vi "Example - Building a Source Distribution.vi"() -> ()   [LabVIEW 2020]
doc: "Demonstrates the use of the Application Builder API to create and build a Source Distribution build specification."
uses:
  <vilib>/AppBuilder/AB_API/common/AB_API Version Number.ctl
  <vilib>/AppBuilder/AB_API/SDIST/NI_AB_API_SDIST.lvclass
panel:
  out "Generated Files":path[](array[path])
  # "Overview: Demonstrates the use of the Application Builder API to create and build a Source Distribution build specification.\nRequirements: LabVIEW Professional Development System or LabVIEW Application Builder\nInstructions:\n1. Run the VI. A Source Distribution build specification will be created, which will then be built programmatically.\n2. Examine the SDIST build specification in the new project.\n3. Close the temporary project and delete the temporary project files generated by this example when you are done."
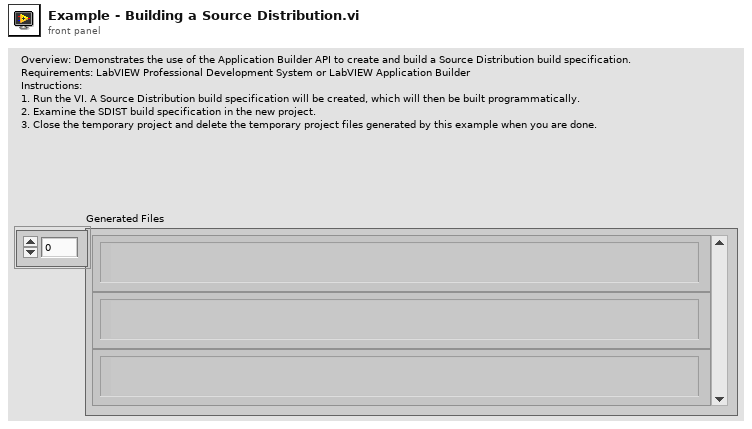
[diagram p1: front panel]
types:
  T1 = typedef "AB_API Version Number.ctl" = cluster{"Major":u16, "Minor":u16, "Fix":u16, "Build":u16}
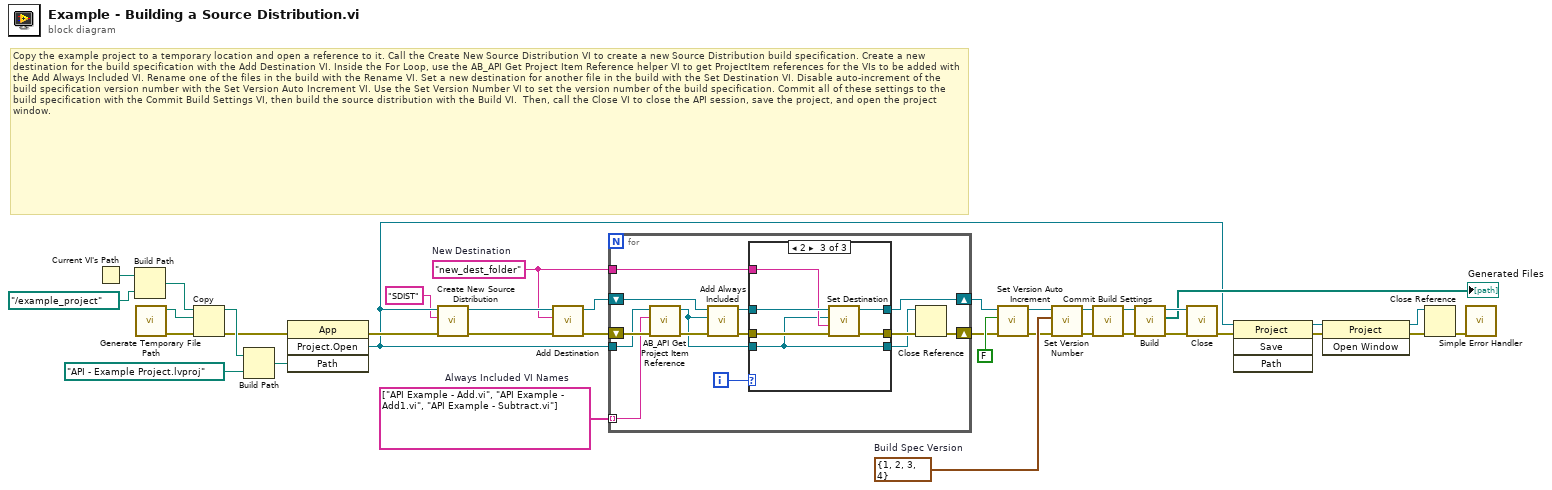
[diagram p0: block diagram]
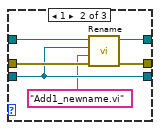
[diagram p3: hidden frame]
diagram:
  w4 = "new_dest_folder"  # New Destination
  w15 = T1 {"Major"=1, "Minor"=2, "Fix"=3, "Build"=4}  # Build Spec Version
  w31 = string[] ["API Example - Add.vi", "API Example - Add1.vi", "API Example - Subtract.vi"]  # Always Included VI Names
  # "Copy the example project to a temporary location and open a reference to it. Call the Create New Source Distribution VI to create a new Source Distribution build specification. Create a new destination for the build specification with the Add Destination VI. Inside the For Loop, use the AB_API Get Project Item Reference helper VI to get ProjectItem references for the VIs to be added with the Add Always Included VI. Rename one of the files in the build with the Rename VI. Set a new destination for another file in the build with the Set Destination VI. Disable auto-increment of the build specification version number with the Set Version Auto Increment VI. Use the Set Version Number VI to set the version number of the build specification. Commit all of these settings to the build specification with the Commit Build Settings VI, then build the source distribution with the Build VI.  Then, call the Close VI to close the API session, save the project, and open the project window."
  n1 = Current VI's Path() -> (path=w30:path)
  n2 = Build Path(base path=w30, name or relative path=path "../example_project" ("path")) -> (appended path=w26:path)
  n3 = call <vilib>:"Generate Temporary File Path.vi"() -> ("error out"=w19:errorcluster, "Unique Temporary File Path"=w25:path)  [unwired: 10 in]
  n4 = Copy(8:w19, 10:w25, 11:w26) -> (0:w18:errorcluster, 3:w24:path)  [unwired: 2 in, 1 out]
  n5 = Build Path(base path=w24, name or relative path=path "API - Example Project.lvproj") -> (appended path=w22:path)
  n6 = invoke class="App" method="Project.Open"(error in=w18, "Path"=w22) -> (error out=w29:errorcluster, "Project:Open"=w21:refnum<vi>)  [unwired: 2 in, 2 out]
  n7 = call <vilib>:"Create New Source Distribution.vi"("error in (no error)"=w29, "Build specification name"="SDIST", "Project Refnum"=w21) -> ("error out"=w17:errorcluster, "SDIST out"=w6:refnum<class "NI_AB_API_SDIST.lvclass">)  [unwired: 7 in]
  n8 = call-dynamic "Add Destination.vi"("error in (no error)"=w17, "Destination label"=w4, "SDIST in"=w6) -> ("error out"=w7:errorcluster, "SDIST out"=w5:refnum<class "NI_AB_API_SDIST.lvclass">)  [unwired: 7 in]
  n9 = for {
    shift-right: [w39] -> w11
    shift-left: w5 -> [w47]
    shift-right: [w51] -> w10
    shift-left: w7 -> [w50]
    tunnel: w21 -> [w49]
    tunnel: w31 -> [w48] mode=indexing
    tunnel: w4 -> [w38]
    i -> [w45]
    n10 = call <vilib>:"AB_API Get Project Item Reference.vi"("error in (no error)"=w50, "Name"=w48, "Project Refnum"=w49) -> ("error out"=w46:errorcluster, "ProjectItem Refnum"=w42:refnum<vi>)  [unwired: 6 in, 1 out]
    n11 = call-dynamic "Add Always Included.vi"("error in (no error)"=w46, "ProjectItem Refnum"=w42, "SDIST in"=w47) -> ("error out"=w44:errorcluster, "SDIST out"=w43:refnum<class "NI_AB_API_SDIST.lvclass">)  [unwired: 7 in]
    n12 = case shown="2" w45 {
      tunnel: w44 -> [w54 w59 w66]
      tunnel: w43 -> [w52 w58 w63]
      tunnel: w42 -> [w53 w56 w61]
      tunnel: [w54 w60 w65] -> w41
      tunnel: [w53 w56 w61] -> w40
      tunnel: [w52 w57 w64] -> w39
      tunnel: w38 -> [_ _ w62]
      frame Default {
      }
      frame 1 {
        n13 = call-dynamic "Rename.vi"("error in (no error)"=w59, "New name"="Add1_newname.vi", "ProjectItem Refnum"=w56, "SDIST in"=w58) -> ("error out"=w60:errorcluster, "SDIST out"=w57:refnum<class "NI_AB_API_SDIST.lvclass">)  [unwired: 6 in]
      }
      frame 2 {
        n14 = call-dynamic "Set Destination.vi"("error in (no error)"=w66, "Destination label"=w62, "ProjectItem Refnum"=w61, "SDIST in"=w63) -> ("error out"=w65:errorcluster, "SDIST out"=w64:refnum<class "NI_AB_API_SDIST.lvclass">)  [unwired: 6 in]
      }
    }
    n15 = Close Reference(reference=w40, error in (no error)=w41) -> (error out=w51:errorcluster)
  }
  n16 = call-dynamic "Set Version Auto Increment.vi"("error in (no error)"=w10, "Auto Increment Version"=FALSE, "NI_AB_API_SDIST in"=w11) -> ("error out"=w14:errorcluster, "NI_AB_API_SDIST out"=w13:refnum<class "NI_AB_API_SDIST.lvclass">)  [unwired: 7 in]
  n17 = call-dynamic "Set Version Number.vi"("error in (no error)"=w14, "Version number"=w15, "SDIST in"=w13) -> ("error out"=w9:errorcluster, "SDIST out"=w8:refnum<class "NI_AB_API_SDIST.lvclass">)  [unwired: 7 in]
  n18 = call-dynamic "Commit Build Settings.vi"("error in (no error)"=w9, "SDIST in"=w8) -> ("error out"=w37:errorcluster, "SDIST out"=w36:refnum<class "NI_AB_API_SDIST.lvclass">)  [unwired: 8 in]
  n19 = call-dynamic "Build.vi"("error in (no error)"=w37, "SDIST in"=w36) -> ("error out"=w34:errorcluster, "GeneratedFiles"=→"Generated Files":path[], "SDIST out"=w35:refnum<class "NI_AB_API_SDIST.lvclass">)  [unwired: 6 in, 1 out]
  n20 = call-dynamic "Close.vi"("error in (no error)"=w34, "SDIST in"=w35) -> ("error out"=w32:errorcluster)  [unwired: 9 in]
  n21 = invoke class="Project" method="Save"(reference=w21, error in=w32) -> (reference out=w2:refnum<vi>, error out=w33:errorcluster)  [unwired: 2 in, 2 out]
  n22 = invoke class="Project" method="Open Window"(reference=w2, error in=w33) -> (reference out=w1:refnum<vi>, error out=w3:errorcluster)  [unwired: 1 in, 1 out]
  n23 = Close Reference(reference=w1, error in (no error)=w3) -> (error out=w28:errorcluster)
  n24 = call <vilib>:"Simple Error Handler.vi"("error in (no error)"=w28) -> ()  [unwired: 4 in, 5 out]
